vi "test.vi"(7 "error in":errorcluster) -> (27 "error out":errorcluster)   [LabVIEW 2018]
uses:
  <vilib>/vision/NI_Vision_Development_Module.lvlib
panel:
  out "Image Out":T1(plugin-control)
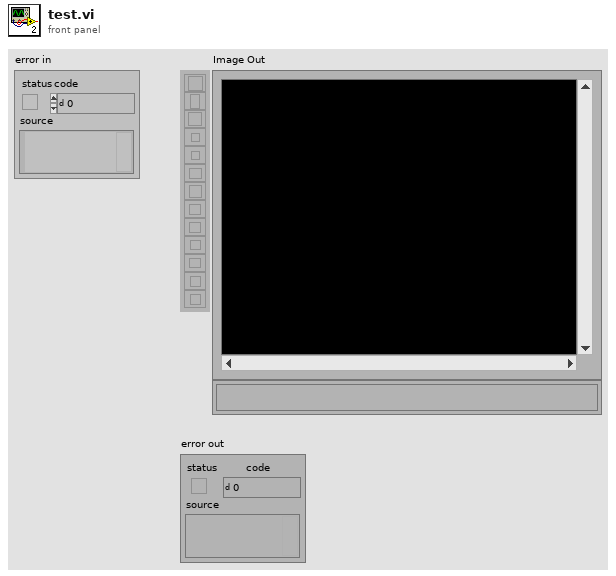
[diagram p1: front panel]
types:
  T1 = typedef "IMAQ Image.ctl" = refnum<image>
  T2 = enum32{"AutoM", "Close", "Dilate", "Erode", "Gradient", "Gradient out", "Gradient in", "Hit miss", "Open", "PClose", "POpen", "Thick", "Thin"}
  T3 = enum32{"AutoM", "Close", "Dilate", "Erode", "Gradient", "Gradient in", "Gradient out", "HitMiss", "Open", "PClose", "POpen", "Thick", "Thin"}
  T4 = cluster{"Global Rectangle":i32[], "Contours":cluster{"ID":enum32{"External", "Internal"}, "Type":u32, "Coordinates":i32[]}[]}
  T5 = typedef "Image Type" = u32
  T6 = cluster{"Pos. X":i32, "Pos. Y":i32, "Radius":i32, "Core Area":i32}[]
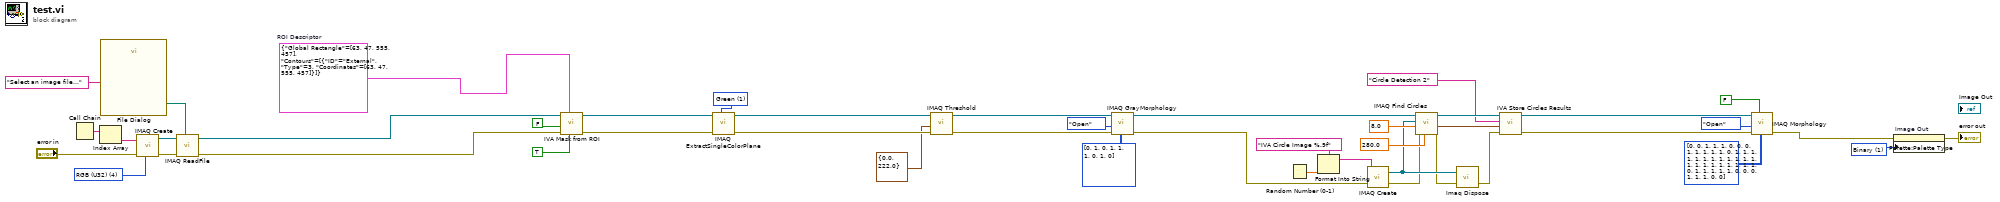
[diagram p0: block diagram]
diagram:
  w1 = u32 1 items=["Grayscale", "Binary", "Gradient", "Rainbow", "Temperature", "User Defined", "Binary 16 Bit", "Gradient 16 Bit", "Rainbow 16 Bit", "Temperature 16 Bit", "User Defined 16 Bit"] ("Palette Type")
  w30 = 1 items=["Red", "Green", "Blue", "Hue", "Saturation", "Luminance", "Value", "Intensity"] ("Color Plane")
  w35 = T4 {"Global Rectangle"=[63, 47, 555, 457], "Contours"=[{"ID"=enum."External", "Type"=3, "Coordinates"=[63, 47, 555, 457]}]}  # ROI Descriptor
  w36 = T5 4 items=["Grayscale (U8)", "Grayscale (I16)", "Grayscale (SGL)", "Complex (CSG)", "RGB (U32)", "HSL (U32)", "RGB (U64)", "Grayscale (U16)"] ("Image Type")
  n1 = Call Chain() -> (call chain=w40:string[])
  n2 = Index Array(array=w40) -> (element=w39:string)  [unwired: 1 in]
  n3 = call "File Dialog"("prompt"="Select an image file...") -> ("selected path"=w37:path)  [unwired: 6 in, 8 out]
  n4 = call "IMAQ Create"("Image Name"=w39, "Image Type"=w36, "error in (no error)"="error in") -> ("New Image"=w43:T1, "error out"=w42:errorcluster)  [unwired: 1 in, 1 out]
  n5 = call "IMAQ ReadFile"("File Path"=w37, "error in (no error)"=w42, "Image"=w43) -> ("error out"=w44:errorcluster, "Image Out"=w33:T1)  [unwired: 2 in, 5 out]
  n6 = call <vilib>:"IVA Mask from ROI.vi"("Shrink"=TRUE, "ROI Descriptor"=w35, "error in (no error)"=w44, "Out / In"=FALSE, "Image Src"=w33) -> ("error out"=w31:errorcluster, "Image Out"=w29:T1)  [unwired: 5 out]
  n7 = call "IMAQ ExtractSingleColorPlane"("Color Plane"=w30, "error in (no error)"=w31, "Image Src"=w29) -> ("error out"=w28:errorcluster, "Image Dst Out"=w26:T1)  [unwired: 1 in, 6 out]
  n8 = call "IMAQ Threshold"("error in (no error)"=w28, "Range"=cluster{"Lower value":sgl, "Upper value":sgl} {"Lower value"=0.0, "Upper value"=222.0}, "Image Src"=w26) -> ("error out"=w25:errorcluster, "Image Dst Out"=w22:T1)  [unwired: 3 in, 4 out]
  n9 = call "IMAQ GrayMorphology"("Structuring Element"=i32[][] [[0, 1, 0], [1, 1, 1], [0, 1, 0]], "error in (no error)"=w25, "Operation"=T3."Open", "Image Src"=w22) -> ("error out"=w21:errorcluster, "Image Dst Out"=w13:T1)  [unwired: 3 in, 3 out]
  n10 = Random Number (0-1)() -> (number: 0 to 1=w8:dbl)
  n11 = Format Into String(format string="IVA Circle Image %.9f" ("Image Name"), w8) -> (resulting string=w10:string)  [unwired: 2 in, 1 out]
  n12 = call "IMAQ Create"("Image Name"=w10, "error in (no error)"=w21) -> ("New Image"=w18:T1, "error out"=w17:errorcluster)  [unwired: 2 in, 1 out]
  n13 = call "IMAQ Find Circles"("Max Radius"=sgl 280.0, "error in (no error)"=w17, "Min Radius"=sgl 8.0, "Image Dst"=w18, "Image Src"=w13) -> ("error out"=w16:errorcluster, "Circles Data"=w11:T6)  [unwired: 5 out]
  n14 = call "Imaq Dispose"("Image"=w18, "error in (no error)"=w16) -> ("error out"=w15:errorcluster)  [unwired: 1 in, 3 out]
  n15 = call <vilib>:"IVA Store Circles Results.vi"("error in (no error)"=w15, "Circles Data"=w11, "Step Name"="Circle Detection 2", "Image in"=w13) -> ("error out"=w14:errorcluster, "Image dup"=w4:T1)  [unwired: 6 out]
  n16 = call "IMAQ Morphology"("Structuring Element"=i32[][] [[0, 0, 1, 1, 1, 0, 0], [0, 1, 1, 1, 1, 1, 0], [1, 1, 1, 1, 1, 1, 1], [1, 1, 1, 1, 1, 1, 1], [1, 1, 1, 1, 1, 1, 1], [0, 1, 1, 1, 1, 1, 0], [0, 0, 1, 1, 1, 0, 0]], "Square/Hexa (Square)"=FALSE, "error in (no error)"=w14, "Operation"=T2."Open", "Image Src"=w4) -> ("error out"=w3:errorcluster)  [unwired: 2 in, 4 out]
  n17 = property on="Image Out" class="ImageControl"(error in=w3, "Palette:Palette Type"=w1) -> (error out=→"error out":errorcluster)  [unwired: 1 in, 1 out]
